vi "X_transfer_Z.vi"(4 "x":dbl format="%#_13g") -> (1 "y":dbl)   [LabVIEW 2015]
panel:
  in  "Xd":dbl[](array[numeric])=[1.0, -0.499999999999867] format="%#_13g"
  in  "Xn":dbl[](array[numeric])=[0.0, 1236.880570776381] format="%#_13g"
  out "yk chain":dbl[](array[numeric])
  out "xk chain":dbl[](array[numeric])
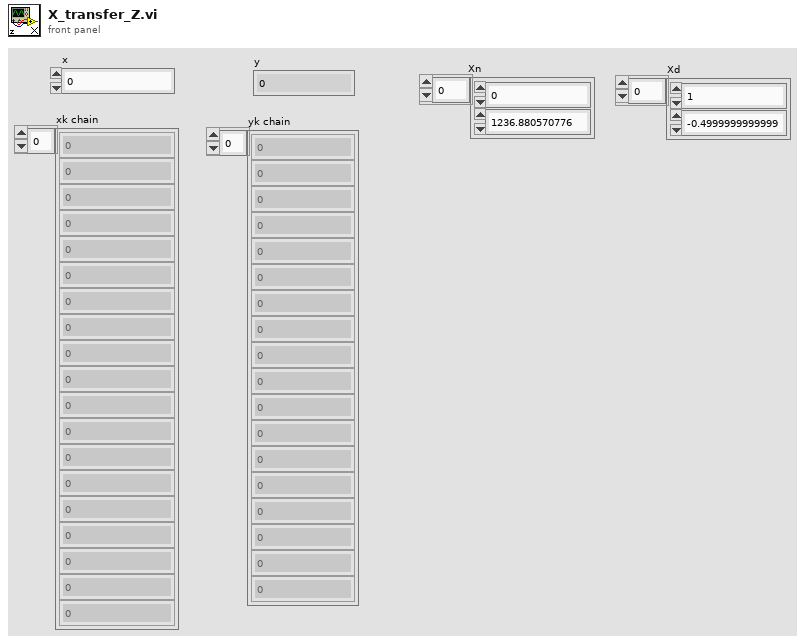
[diagram p1: front panel]
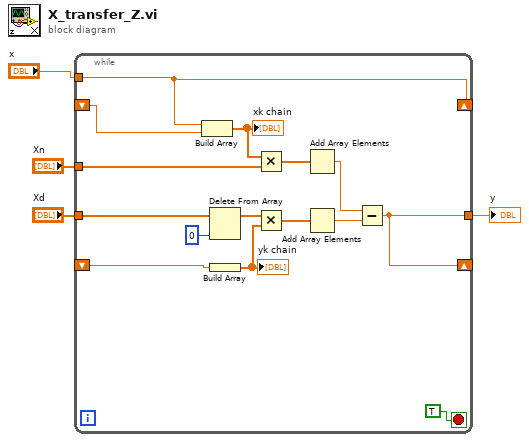
[diagram p0: block diagram]
diagram:
  n1 = while {
    tunnel: [w6] -> w4
    tunnel: "x" -> [w8]
    tunnel: "Xd" -> [w10]
    tunnel: "Xn" -> [w11]
    shift-right: [w8] -> _
    shift-left: _ -> [w7]
    shift-right: [w6] -> _
    shift-left: _ -> [w5]
    stop <- TRUE stop-if-true
    n2 = Build Array(w8, w7) -> (w12:dbl[])
    "xk chain" <- w12
    n3 = Delete From Array(array=w10, index=0) -> (array with subset deleted=w16:dbl[])  [unwired: 1 in, 1 out]
    n4 = Build Array(w5) -> (w9:dbl[])
    "yk chain" <- w9
    n5 = Multiply(x=w12, y=w11) -> (x*y=w19:dbl[])
    n6 = Multiply(x=w16, y=w9) -> (x*y=w17:dbl[])
    n7 = Add Array Elements(numeric array=w19) -> (sum=w15:dbl)
    n8 = Add Array Elements(numeric array=w17) -> (sum=w14:dbl)
    n9 = Subtract(x=w15, y=w14) -> (x-y=w6:dbl)
  }
  "y" <- w4
